vi "Configure OPP State and Level.vi"(7 "State":bool, 8 "error in":errorcluster, 9 "OPP Delay(S)":dbl min=0.0 max=10.0, 10 "OPP Level(W)":dbl min=0.0 max=860.0, 11 "VISA resource name":refnum<visa-resource-name>) -> (0 "error out":errorcluster, 3 "VISA resource name out":refnum<visa-resource-name>)   [LabVIEW 2018, in "IT-M3100.lvlib"]
doc: "The command to configure whether to enable OPP, over power protection Level and over power protection delay time.\n<b>OPP Level(W)</b>\n0-860\n<b>OPP Delay(S)</b>\n0-10"
uses:
  IT-M3100.lvlib
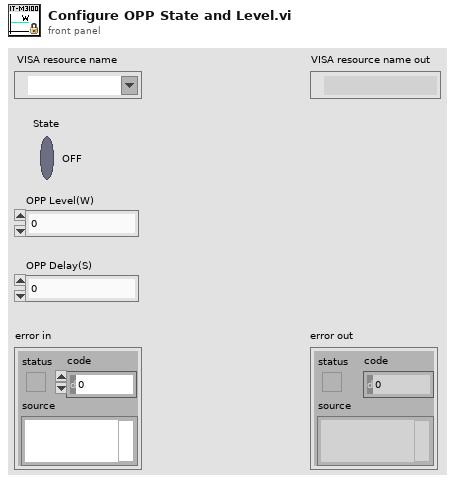
[diagram p1: front panel]
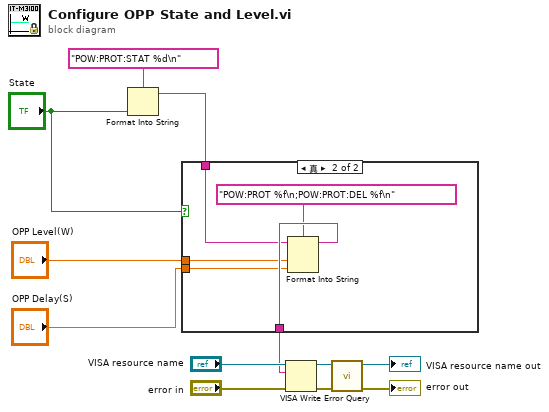
[diagram p0: block diagram]
diagram:
  n1 = Format Into String(format string="POW:PROT:STAT %d\n", "State") -> (resulting string=w4:string)  [unwired: 2 in, 1 out]
  n2 = case shown="真" "State" {
    tunnel: w4 -> [w13 w16]
    tunnel: [w13 w18] -> w5
    tunnel: "OPP Level(W)" -> [_ w15]
    tunnel: "OPP Delay(S)" -> [_ w14]
    frame False {
    }
    frame True {
      n3 = Format Into String(format string="POW:PROT %f\n;POW:PROT:DEL %f\n", initial string=w16, w15, w14) -> (resulting string=w18:string)  [unwired: 1 in, 1 out]
    }
  }
  n4 = VISA Write(VISA resource name="VISA resource name", write buffer=w5, error in (no error)="error in") -> (VISA resource name out=w9:refnum<visa-resource-name>, error out=w10:errorcluster)  [unwired: 1 out]
  n5 = call "Error Query.vi"("error in"=w10, "VISA resource name"=w9) -> ("error out"=→"error out":errorcluster, "VISA resource name out"=→"VISA resource name out":refnum<visa-resource-name>)  [unwired: 6 in, 2 out]
